vi "Lab 2 Part A.vi"() -> ()   [LabVIEW 2020]
uses:
  <vilib>/MakerHub/LINX/Public/Utilities/Open Serial.vi
  <vilib>/addons/control/pid/pid.llb/PID (DBL).vi
  <vilib>/addons/control/pid/NI_PID_pid.lvlib
  <vilib>/MakerHub/LINX/LMH-LINX.lvlib
panel:
  out "Duty Cycle":dbl
  in  "output range":cluster{"output high":dbl, "output low":dbl}={"output high"=100.0, "output low"=-100.0} {"output low" format="%.2f"; "output high" format="%.2f"}
  out "Output Chart":dynamicdata(graph)
  in  "PID gains":T1={"proportional gain (Kc)"=6.0, "integral time (Ti, min)"=0.003, "derivative time (Td, min)"=0.0001} {"derivative time (Td, min)" format="%.6f"; "integral time (Ti, min)" format="%.6f"; "proportional gain (Kc)" format="%.3f"}
  out "Voltage":dbl
  in  "Stop Button":bool
  in  "PWM Channel":u8=10
  in  "AI1 and AI2 Channels":u8[](array[numeric])
  in  "Hall Channel":u8
  in  "Serial Port":refnum<visa-resource-name>="N/A"
  in  "Set Point":dbl
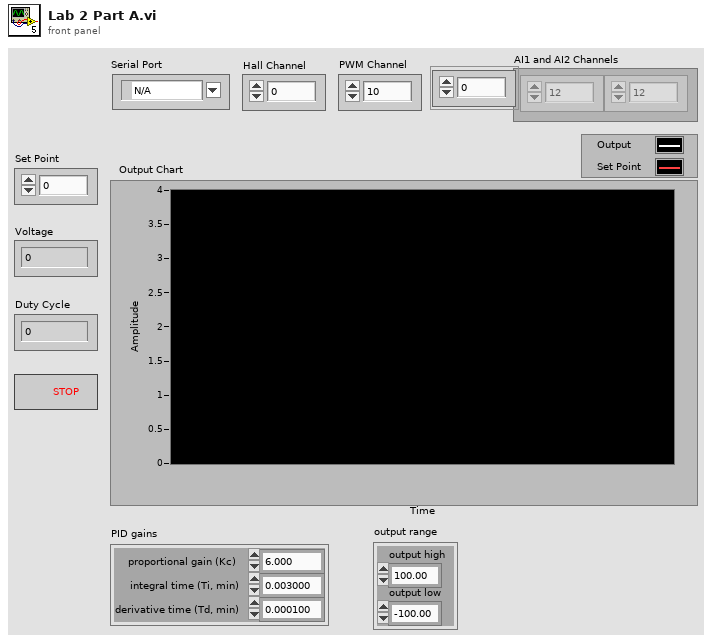
[diagram p1: front panel]
types:
  T1 = cluster{"proportional gain (Kc)":dbl, "integral time (Ti, min)":dbl, "derivative time (Td, min)":dbl}
  T2 = typedef "LMH-LINX.lvlib/LINX Ref.ctl" = cluster{"IO":T3, "Interface":T4, "LINX Device Config":T5}
  T3 = typedef "LMH-LINX.lvlib/Platform.ctl" = enum16{"Remote", "Local"}
  T4 = typedef "LMH-LINX.lvlib/Interface.ctl" = enum16{"Serial", "TCP"}
  T5 = typedef "LMH-LINX.lvlib/Device.lvlib/LINX Device Config.ctl" = cluster{"Interface":T4, "COM Port":refnum<visa-resource-name>, "TCP Configuration":T6, "Device Family":u8, "Device ID":u8, "Device Name":string, "TCP Ref":refnum<k5>, "Channels":T7}
  T6 = typedef "LMH-LINX.lvlib/Device.lvlib/TCP Config.ctl" = cluster{"IP Address":string, "Port":u16}
  T7 = typedef "LMH-LINX.lvlib/Channels.ctl" = cluster{"DI":u8[], "DO":u8[], "AI":u8[], "AO":u8[], "PWM":u8[], "QE":u8[], "UART":u8[], "I2C 2":u8[], "SPI":u8[], "CAN":u8[], "Servo":u8[], "AI Ref (V)":dbl, "AI Resolution (Bits)":u8, "AO Ref (V)":dbl, "AO Resolution (Bits)":u8}
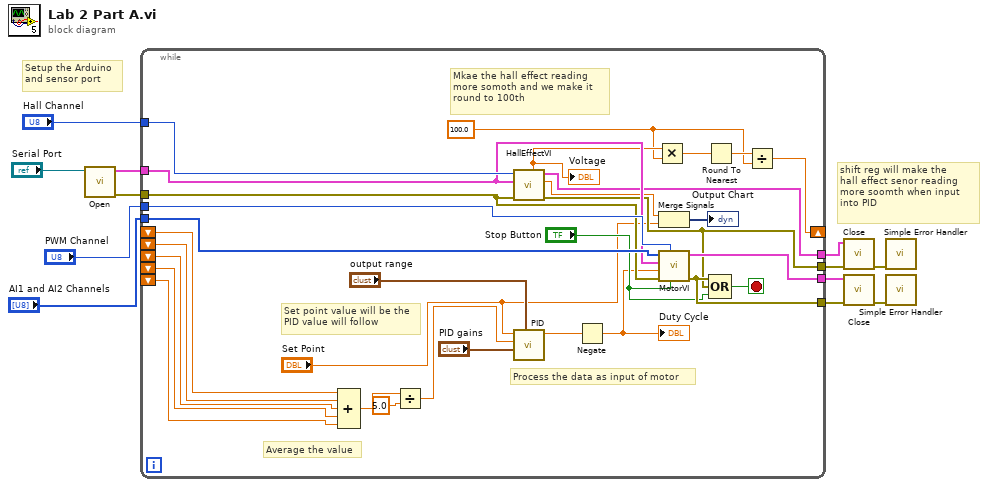
[diagram p0: block diagram]
diagram:
  # "shift reg will make the\nhall effect senor reading\nmore soomth when input \ninto PID"
  # "Setup the Arduino\nand sensor port"
  n1 = call-poly <vilib>:"Open.vi"("Serial Port"="Serial Port") -> ("Error Out"=w7:errorcluster, "LINX Resource"=w8:T2)  [unwired: 8 in, 1 out]
  n2 = while {
    tunnel: "Hall Channel" -> [w43]
    tunnel: "AI1 and AI2 Channels" -> [w42]
    tunnel: "PWM Channel" -> [w41]
    tunnel: w8 -> [w40]
    tunnel: w7 -> [w35]
    tunnel: [w37] -> w6
    tunnel: [w36] -> w5
    tunnel: [w34] -> w4
    tunnel: [w33] -> w3
    shift-right: [w16] -> _
    shift-left: _ -> [w30]
    shift-left: _ -> [w29]
    shift-left: _ -> [w28]
    shift-left: _ -> [w27]
    shift-left: _ -> [w22]
    stop <- w31 stop-if-true
    w17 = 100.0 ("y")
    # "Process the data as input of motor"
    # "Mkae the hall effect reading\nmore somoth and we make it\nround to 100th"
    # "Set point value will be the\nPID value will follow"
    # "Average the value"
    n3 = Compound Arithmetic op=ADD(w30, w29, w28, w27, w22) -> (w26:dbl)
    n4 = Divide(x=w26, y=5.0) -> (x/y=w21:dbl)
    n5 = call "HallEffectVI.vi"("error in (no error)"=w35, "LINX Resource in"=w40, "Analog Channel"=w43) -> ("error out"=w33:errorcluster, "Waveform Chart"=w15:dbl, "LINX Resource out"=w36:T2, "Voltage"=w20:dbl)  [unwired: 5 in]
    "Voltage" <- w20
    n6 = call-poly <vilib>:"PID.vi"("output range"="output range", "PID gains"="PID gains", "process variable"=w21, "setpoint"="Set Point") -> ("output"=w23:dbl)  [unwired: 6 in, 1 out]
    n7 = Negate(x=w23) -> (-x=w24:dbl)
    "Duty Cycle" <- w24
    n8 = Multiply(x=w20, y=w17) -> (x*y=w19:dbl)
    n9 = Merge Signals(w15, "Set Point") -> (→"Output Chart":dynamicdata)
    n10 = call "MotorVI.vi"("stop"="Stop Button", "PWM Channel"=w41, "error in (no error)"=w35, "Duty Cycle (-100 to +100)"=w24, "LINX Resource in"=w40, "AI1 and AI2 Channels"=w42) -> ("error out"=w34:errorcluster, "LINX Resource out"=w37:T2)  [unwired: 3 in, 1 out]
    n11 = Round To Nearest(number=w19) -> (nearest integer value=w18:dbl)
    n12 = Compound Arithmetic op=OR(w34, w33, "Stop Button") -> (w31:bool)
    n13 = Divide(x=w18, y=w17) -> (x/y=w16:dbl)
  }
  n14 = call <vilib>:"Close.vi"("Error In"=w3, "LINX Resource"=w5) -> ("Error Out"=w1:errorcluster)  [unwired: 9 in]
  n15 = call <vilib>:"Close.vi"("Error In"=w4, "LINX Resource"=w6) -> ("Error Out"=w2:errorcluster)  [unwired: 9 in]
  n16 = call <vilib>:"Simple Error Handler.vi"("error in (no error)"=w1) -> ()  [unwired: 4 in, 5 out]
  n17 = call <vilib>:"Simple Error Handler.vi"("error in (no error)"=w2) -> ()  [unwired: 4 in, 5 out]
